vi "CmdexPwmCmd.vi"(0 "Error Input":errorcluster, 5 "PWM Id":enum16{"PWM0", "PWM1", "PWM2", "PWM3"}(ring), 7 "PWM Comd":T1(ring), 9 "Data":sgl=50.0, 11 "Uart Input":cluster{u64} {"?" format="%x"}) -> (4 "Error Output":errorcluster, 15 "Uart Output":cluster{u64} {"?" format="%x"})   [LabVIEW 2019]
doc: "<B>Cmdex</B>\nSends a command to the PWM controller."
uses:
  dll/LabViewUart.dll
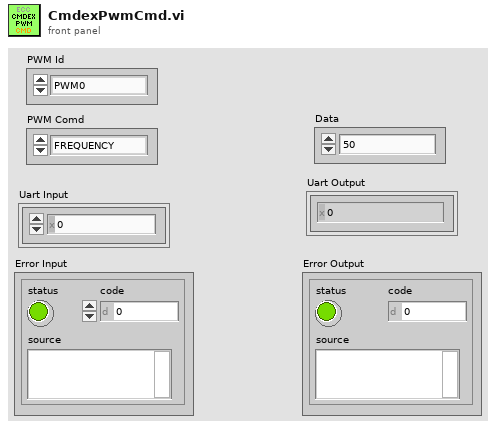
[diagram p1: front panel]
types:
  T1 = enum16{"FREQUENCY", "DUTY RATIO", "PHASE SHIFT", "STOP/START"}
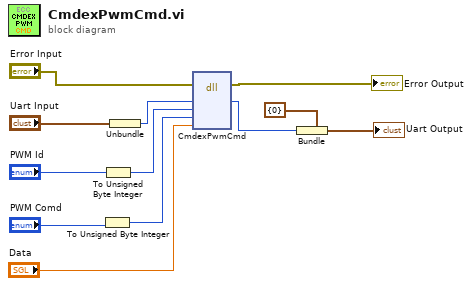
[diagram p0: block diagram]
diagram:
  n1 = To Unsigned Byte Integer(number="PWM Comd") -> (unsigned 8bit integer=w5:u8)
  n2 = To Unsigned Byte Integer(number="PWM Id") -> (unsigned 8bit integer=w7:u8)
  n3 = Unbundle("Uart Input") -> (w9:u64)
  n4 = dll-call lib="D:/Google Drive/INC-2020/INC352/INC352-2020/LabVIEW/examples/uart-cmdex/SubVI/dll/LabViewUart.dll" fn="CmdexPwmCmd"(error in="Error Input", "Uart Handle"=w9, "id"=w7, "cmd"=w5, "data"="Data") -> (error out=→"Error Output":errorcluster, "Uart Handle"=w2:u64)  [unwired: 6 in, 1 out]
  n5 = Bundle(cluster=cluster{u64} {0}, w2) -> (→"Uart Output":cluster{u64})
